vi "PXI-Set 24-bit Board Terminal Config.vi"(11 "error in (no error)":errorcluster) -> (15 "error out":errorcluster)   [LabVIEW 2020]
uses:
  <vilib>/DAQmx/write.llb/DAQmx Write (Analog 2D DBL NChan NSamp).vi
  <vilib>/DAQmx/create/channels.llb/DAQmx Create Channel (AO-Voltage-Basic).vi
  <vilib>/DAQmx/configure/timing.llb/DAQmx Timing (Sample Clock).vi
  <vilib>/DAQmx/miscellaneous.llb/DAQmx Fill In Error Info.vi
  <resource>/objmgr/daqmx.rc
panel:
  in  "output terminal configuration":i32(ring)=12529 items=["Default"=-1, "RSE"=10083, "Differential"=10106, "Pseudodifferential"=12529]
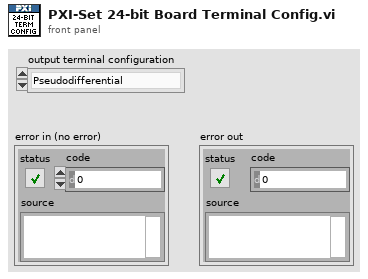
[diagram p1: front panel]
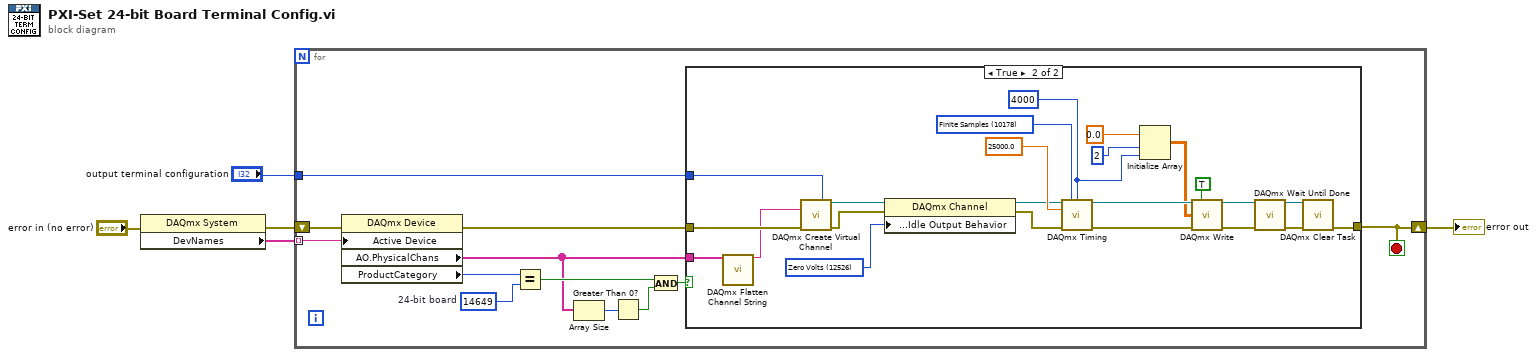
[diagram p0: block diagram]
diagram:
  n1 = property class="DAQmx System"(error in="error in (no error)") -> (error out=w5:errorcluster, "DevNames"=w4:tag[])  [unwired: 1 in, 1 out]
  n2 = for {
    tunnel: w4 -> [w16] mode=indexing
    shift-right: [w11] -> w2
    shift-left: w5 -> [w17]
    tunnel: "output terminal configuration" -> [w10]
    stop <- w11 stop-if-true
    w15 = 14649  # 24-bit board
    n3 = property class="DAQmx Device"(error in=w17, "Active Device"=w16) -> (error out=w12:errorcluster, "AO.PhysicalChans"=w9:tag[], "ProductCategory"=w14:i32)  [unwired: 1 in, 1 out]
    n4 = Equal?(x=w14, y=w15) -> (x = y?=w13:bool)
    n5 = Array Size(array=w9) -> (size(s)=w7:i32)
    n6 = Greater Than 0?(x=w7) -> (x > 0?=w6:bool)
    n7 = And(x=w13, y=w6) -> (x .and. y?=w8:bool)
    n8 = case shown="True" w8 {
      tunnel: w12 -> [w18 w41]
      tunnel: w9 -> [_ w24]
      tunnel: [w18 w27] -> w11
      tunnel: w10 -> [_ w28]
      frame False {
      }
      frame True {
        w23 = 12526 items=["Zero Volts"=12526, "High Impedance"=12527, "Maintain Existing Value"=12528] ("AO.IdleOutputBehavior")
        w39 = 4000 ("samples per channel")
        w30 = 10178 items=["Finite Samples"=10178, "Continuous Samples"=10123, "Hardware Timed Single Point"=12522] ("sample mode")
        n9 = call <vilib>:"DAQmx Flatten Channel String.vi"("names in"=w24) -> ("names out"=w40:string)  [unwired: 13 in, 1 out]
        n10 = call-poly <vilib>:"DAQmx Create Virtual Channel.vi"("output terminal configuration"=w28, "physical channels"=w40, "error in"=w41) -> ("task out"=w22:refnum<k21>, "error out"=w19:errorcluster)  [unwired: 11 in]
        n11 = property class="DAQmx Channel"(reference=w22, error in=w19, "Analog Output:General Properties:Output Configuration:Idle Output Behavior"=w23) -> (reference out=w21:refnum<k21>, error out=w20:errorcluster)
        n12 = call-poly <vilib>:"DAQmx Timing.vi"("task/channels in"=w21, "sample mode"=w30, "samples per channel"=w39, "rate"=25000.0, "error in"=w20) -> ("task out"=w36:refnum<k21>, "error out"=w37:errorcluster)  [unwired: 9 in]
        n13 = Initialize Array(0.0 ("element"), 2 ("dimension size"), w39) -> (w34:dbl[][])
        n14 = call-poly <vilib>:"DAQmx Write.vi"("task/channels in"=w36, "auto start"=TRUE, "data"=w34, "error in"=w37) -> ("task out"=w32:refnum<k21>, "error out"=w33:errorcluster)  [unwired: 9 in, 1 out]
        n15 = call <vilib>:"DAQmx Wait Until Done.vi"("task/channels in"=w32, "error in"=w33) -> ("task out"=w25:refnum<k21>, "error out"=w26:errorcluster)  [unwired: 12 in]
        n16 = call <vilib>:"DAQmx Clear Task.vi"("task in"=w25, "error in"=w26) -> ("error out"=w27:errorcluster)  [unwired: 13 in]
      }
    }
  }
  "error out" <- w2
